vi "Smooth Image by down sample & up sample.vi"(6 "Decimate Factor (2)":i32=2, 8 "error in":errorcluster, 10 "Smoothed Image Dst":T1, 11 "Image to Smooth":T1) -> (0 "error out":errorcluster, 2 "Elapsed time (ms)":u32, 3 "Image Dst Out":T1)   [LabVIEW 2013]
doc: "This vi smooths the input image by down sampling (using decimate factor) then resizing image back to original size.\n\nREENTRANT to allow parallel non blocking calls."
uses:
  <vilib>/vision/Image Controls.llb/IMAQ Image.ctl
  <vilib>/vision/NI_Vision_Development_Module.lvlib
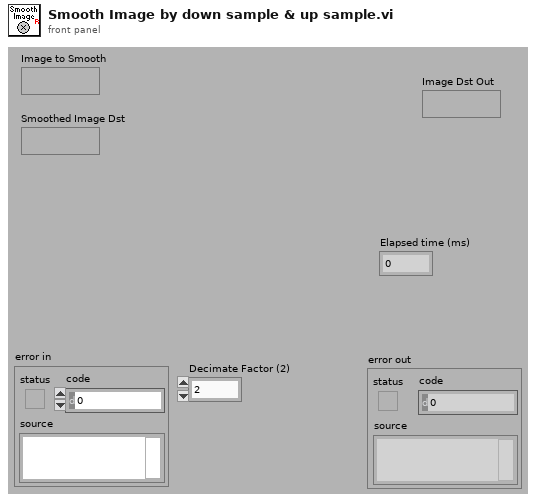
[diagram p1: front panel]
types:
  T1 = typedef "IMAQ Image.ctl" = refnum<image>
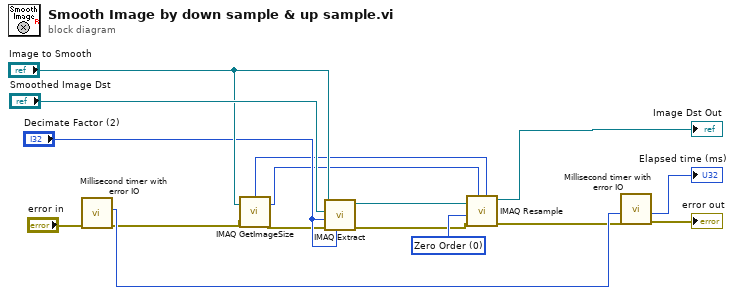
[diagram p0: block diagram]
diagram:
  w4 = u32 0 items=["Zero Order", "Bi-Linear", "Quadratic", "Cubic Spline"] ("Interpolation Type")
  n1 = call "Millisecond timer with error IO.vi"("error in"="error in") -> ("error out"=w3:errorcluster, "current millisecond timer value"=w14:u32)  [unwired: 4 in, 1 out]
  n2 = call "IMAQ GetImageSize"("Image"="Image to Smooth", "error in (no error)"=w3) -> ("Y Resolution"=w5:i32, "X Resolution"=w6:i32, "error out"=w7:errorcluster)  [unwired: 2 in]
  n3 = call "IMAQ Extract"("Y Step Size"="Decimate Factor (2)", "error in (no error)"=w7, "X Step Size"="Decimate Factor (2)", "Image Dst"="Smoothed Image Dst", "Image Src"="Image to Smooth") -> ("error out"=w2:errorcluster, "Image Dst Out"=w1:T1)  [unwired: 5 in]
  n4 = call "IMAQ Resample"("X Resolution"=w6, "Y Resolution"=w5, "error in (no error)"=w2, "Interpolation Type"=w4, "Image Src"=w1) -> ("error out"=w11:errorcluster, "Image Dst Out"=→"Image Dst Out":T1)  [unwired: 5 in]
  n5 = call "Millisecond timer with error IO.vi"("error in"=w11, "T0 time (ms)"=w14) -> ("error out"=→"error out":errorcluster, "Elapsed time (ms)"=→"Elapsed time (ms)":u32)  [unwired: 1 in, 3 out]
